vi "Realsense Cam Frame Process.vi"(4 "Filter settings":T2={"Decimation Scale (1-10)"=3, "Spatial Alpha\n(0-1)"=0.6, "Spatial Delta \n(1/32 disp)"=8, "Temporal Alpha\n(0-1)"=0.4, "Temporal Delta\n(1/32 disp)"=20, "Persistence (0= none, 8=max)"=0, "spatial holefill radius\n(0 disable, 5 max) "=0, "spatial iteration\n(2=default)"=2} {"spatial iteration\n(2=default)" min=1 max=10; "Decimation Scale (1-10)" min=1 max=10; "Spatial Alpha\n(0-1)" min=0 max=1 format="%_2g"; "Spatial Delta \n(1/32 disp)" min=1; "Temporal Alpha\n(0-1)" min=0 max=1 format="%_2g"; "Temporal Delta\n(1/32 disp)" min=1; "Persistence (0= none, 8=max)" max=8; "spatial holefill radius\n(0 disable, 5 max)" max=6}, 5 "Height":i32, 6 "Settings":T1={"Subsample"=TRUE, "Spatial filter"=TRUE, "Temporal filter"=TRUE}, 7 "Width":i32, 8 "error in (no error)":errorcluster, 10 "Frame Data":u64, 11 "Stream type":T3(ring)) -> (0 "error out":errorcluster, 2 "Bytes":u8[](array[numeric]), 3 "Depth":sgl[][](array[numeric]))   [LabVIEW 2018, in "Realsense Cam.lvclass"]
uses:
  Realsense Cam.lvclass
  Temp/realsense_labview_sdk/RealSense SDK2.11.0 for LabVIEW/libRealSense3.lvlib
panel:
  in  "Color format 10":enum16{"Monochrome", "RGB internal (RGB)"}(ring)
  in  "Color format 9":enum16{"Monochrome", "RGB internal (RGB)"}(ring)
  in  "Color format 8":enum16{"Monochrome", "RGB internal (RGB)"}(ring)
  in  "Color format 7":enum16{"Monochrome", "RGB internal (RGB)"}(ring)
  in  "Color format 6":enum16{"Monochrome", "RGB internal (RGB)"}(ring)
  in  "Color format 5":enum16{"Monochrome", "RGB internal (RGB)"}(ring)
  in  "Color format 4":enum16{"Monochrome", "RGB internal (RGB)"}(ring)
  in  "Color format 3":enum16{"Monochrome", "RGB internal (RGB)"}(ring)
  in  "Color format 2":enum16{"Monochrome", "RGB internal (RGB)"}(ring)
  in  "Color format":enum16{"Monochrome", "RGB internal (RGB)"}(ring)
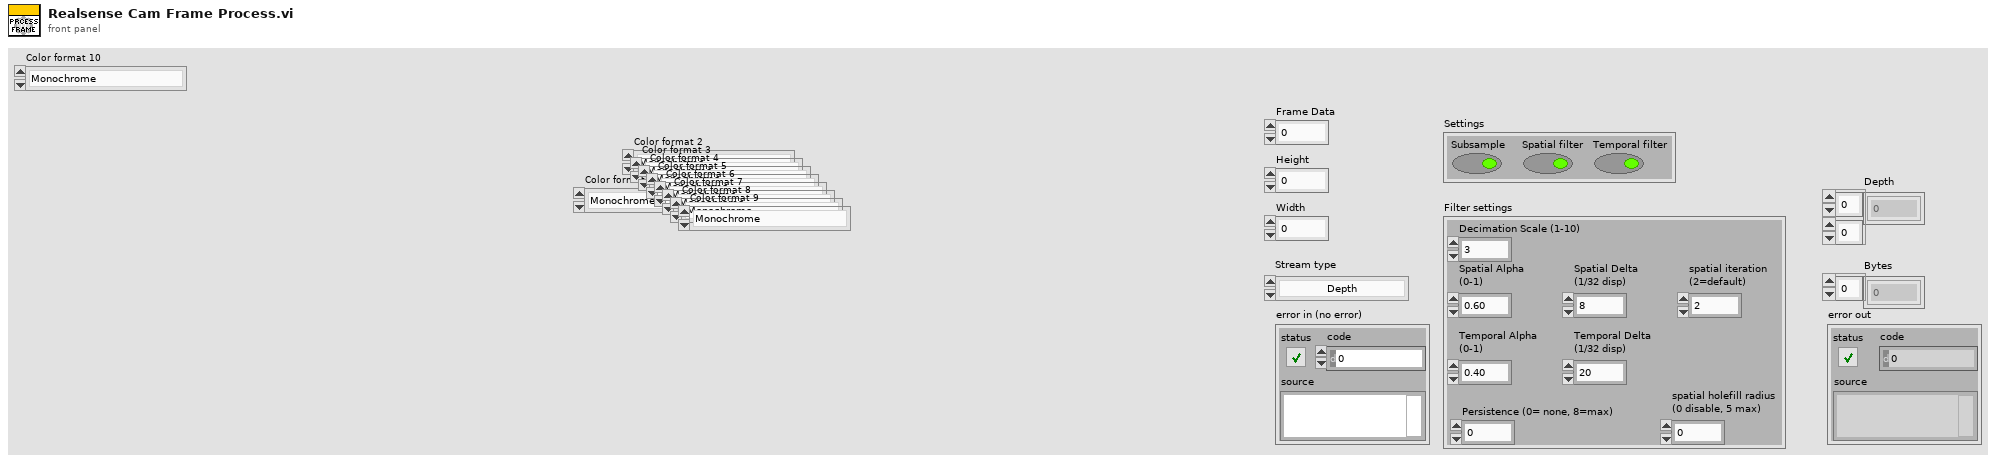
[diagram p1: front panel]
types:
  T1 = cluster{"Subsample":bool, "Spatial filter":bool, "Temporal filter":bool}
  T2 = cluster{"Decimation Scale (1-10)":u8, "Spatial Alpha\n(0-1)":sgl, "Spatial Delta \n(1/32 disp)":u16, "Temporal Alpha\n(0-1)":sgl, "Temporal Delta\n(1/32 disp)":u16, "Persistence (0= none, 8=max)":u8, "spatial holefill radius\n(0 disable, 5 max) ":u8, "spatial iteration\n(2=default)":u8}
  T3 = enum16{"Depth", "Color (ext.)", "Color (left) ", "IR Left", "IR Right", "IR Left (Y16)", "IR Right (Y16)"}
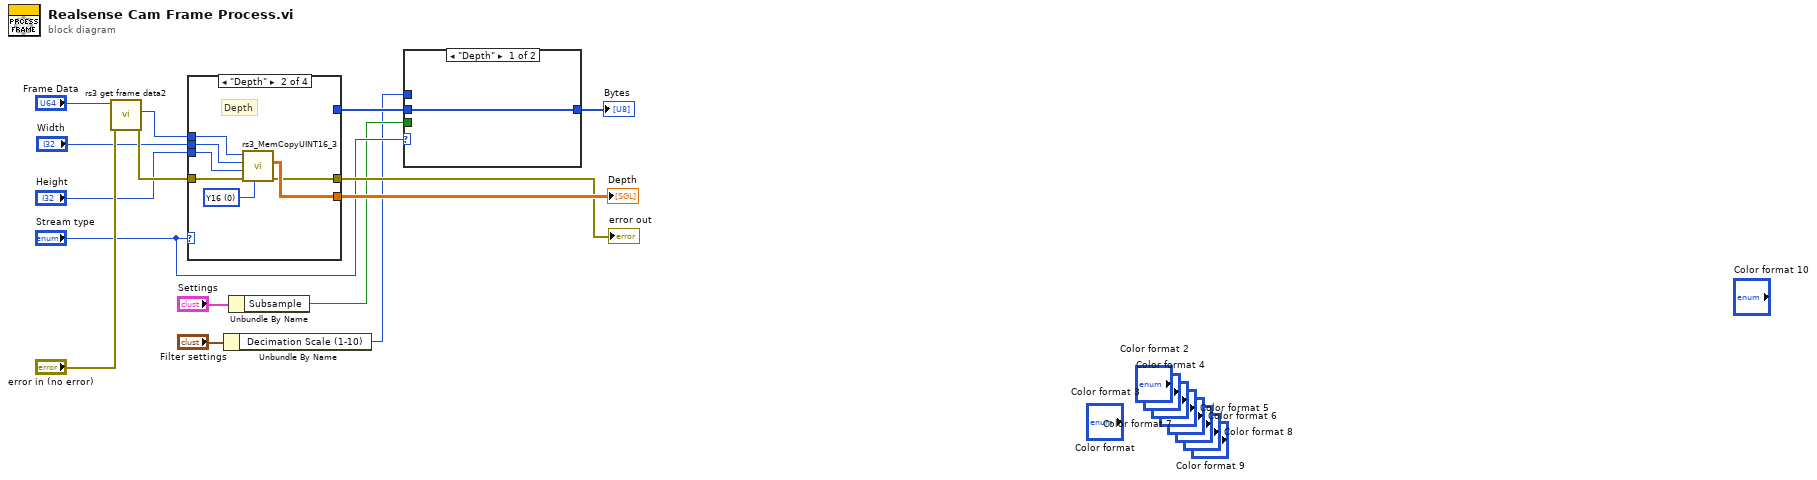
[diagram p0: block diagram]
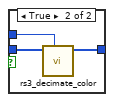
[diagram p3: hidden frame]
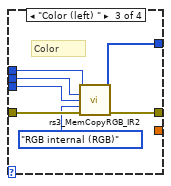
[diagram p5: hidden frame]
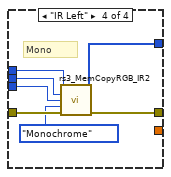
[diagram p6: hidden frame]
diagram:
  n1 = call "rs3 get frame data2.vi"("error in (no error)"="error in (no error)", "frame in"="Frame Data") -> ("error out"=w13:errorcluster, "image pointer out"=w10:u64)  [unwired: 6 in, 2 out]
  n2 = case shown="\"Depth\"" "Stream type" {
    tunnel: [w16 w20 w30 w37] -> w8
    tunnel: w13 -> [w16 w21 w29 w36]
    tunnel: [_ w22 _ _] -> w9
    tunnel: [_ _ w28 w35] -> w6
    tunnel: "Height" -> [_ w19 w24 w31]
    tunnel: "Width" -> [_ w18 w25 w32]
    tunnel: w10 -> [_ w17 w26 w33]
    frame "Color (ext.)", Default {
    }
    frame "Depth" {
      w23 = u16 0 items=["Y16", "Y8"] ("Image format")
      # "Depth"
      n3 = call "rs3_MemCopyUINT16_3.vi"("Image format"=w23, "error in (no error)"=w21, "Depth Y"=w19, "Depth X"=w18, "Zimage pointer"=w17) -> ("error out"=w20:errorcluster, "2D Array Output"=w22:sgl[][])  [unwired: 3 in, 2 out]
    }
    frame "Color (left) " {
      # "Color"
      n4 = call "rs3_MemCopyRGB_IR2.vi"("Zimage pointer"=w26, "RGB  X, width"=w25, "RGB Y, height"=w24, "Color format"=enum16{"Monochrome", "RGB internal (RGB)"}."RGB internal (RGB)", "error in (no error)"=w29) -> ("Output Array"=w28:u8[], "error out"=w30:errorcluster)  [unwired: 8 in, 1 out]
    }
    frame "IR Left" {
      # "Mono"
      n5 = call "rs3_MemCopyRGB_IR2.vi"("Zimage pointer"=w33, "RGB  X, width"=w32, "RGB Y, height"=w31, "Color format"=enum16{"Monochrome", "RGB internal (RGB)"}."Monochrome", "error in (no error)"=w36) -> ("Output Array"=w35:u8[], "error out"=w37:errorcluster)  [unwired: 8 in, 1 out]
    }
  }
  "Depth" <- w9
  "error out" <- w8
  n6 = Unbundle By Name("Filter settings") -> ("Decimation Scale (1-10)"=w1:u8)
  n7 = Unbundle By Name("Settings") -> ("Subsample"=w2:bool)
  n8 = case shown="\"Depth\"" "Stream type" {
    tunnel: w6 -> [w38 w42]
    tunnel: [w38 w41] -> w3
    tunnel: w2 -> [_ w40]
    tunnel: w1 -> [_ w39]
    frame "Depth" {
    }
    frame "Color (ext.)", Default {
      n9 = case shown="False" w40 {
        tunnel: w42 -> [w43 w46]
        tunnel: [w43 w45] -> w41
        tunnel: w39 -> [_ w44]
        frame False {
        }
        frame True {
          n10 = call "rs3_decimate_color.vi"("Decimate"=w44, "input image"=w46) -> ("decimated color"=w45:u8[])  [unwired: 7 in, 2 out]
        }
      }
    }
  }
  "Bytes" <- w3
